vi "LoadPluginRequest.vi"(8 "error in (no error)":errorcluster, 10 "PathToPluginINI":path, 11 "ModuleID":i32) -> (0 "error out":errorcluster)   [LabVIEW 2018, in "SensorModule.lvlib"]
uses:
  SensorModule.lvlib
  SensorShared/clEventType.ctl
  <vilib>/Utility/error.llb/Error Cluster From Error Code.vi
  <vilib>/ErrorRing/Error Ring.xnode
  SensorShared/SensorShared.lvlib
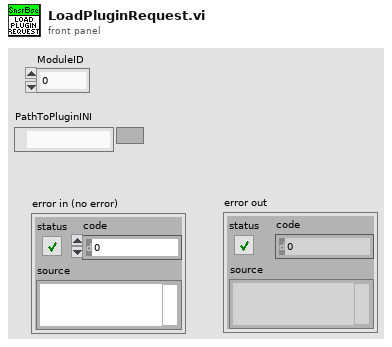
[diagram p1: front panel]
types:
  T1 = typedef "SensorShared.lvlib/clRequestEvents.ctl" = cluster{"StopRequest":refnum<user-event>, "PathToINI":refnum<user-event>, " LoadPlugin":refnum<user-event>, "ShowPanel":refnum<user-event>, "StartData":refnum<user-event>, "StopData":refnum<user-event>, "WriteConfig":refnum<user-event>, "ReadConfig":refnum<user-event>, "WriteEvtSignal":refnum<user-event>, "Configure":refnum<user-event>}
  T2 = typedef "SensorShared.lvlib/clEventType.ctl" = cluster{"ModuleID":i32, "Data":variant}
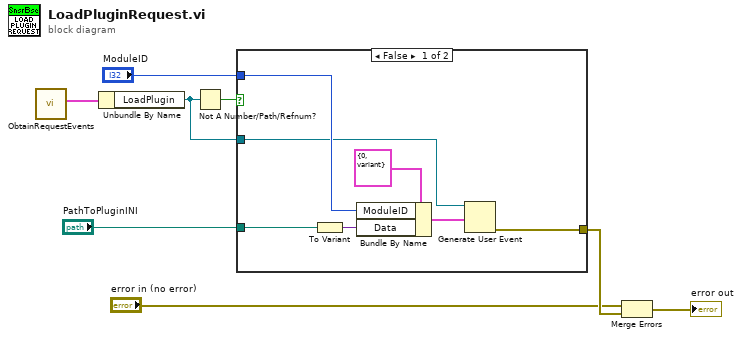
[diagram p0: block diagram]
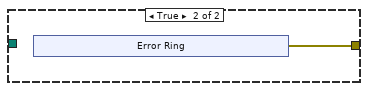
[diagram p2: hidden frame]
diagram:
  n1 = call "ObtainRequestEvents.vi"() -> ("clRequestEvents"=w8:T1)  [unwired: 10 in, 1 out]
  n2 = Unbundle By Name(w8) -> ("LoadPlugin"=w6:refnum<user-event>)
  n3 = Not A Number/Path/Refnum?(number/path/refnum=w6) -> (NaN/Path/Refnum?=w7:bool)
  n4 = case shown="False" w7 {
    tunnel: w6 -> [w12 _]
    tunnel: "ModuleID" -> [w14 _]
    tunnel: [w11 w16] -> w3
    tunnel: "PathToPluginINI" -> [w9 _]
    frame False {
      n5 = To Variant(anything=w9) -> (Variant=w10:variant)
      n6 = Bundle By Name(cluster=T2 {"ModuleID"=0, "Data"=variant} ("clEventType"), "ModuleID"=w14, "Data"=w10) -> (w13:T2)
      n7 = Generate User Event(user event=w12, event data cluster=w13) -> (error out=w11:errorcluster)  [unwired: 2 in, 1 out]
    }
    frame True {
      n8 = xnode "Error Ring"() -> ("error out"=w16:errorcluster)
    }
  }
  n9 = Merge Errors("error in (no error)", w3) -> (→"error out":errorcluster)
